vi "Clear All Disconnected MHLC.vi"(8 "error in (no error)":errorcluster, 10 "Data in":variant, 11 "AppMgr in":refnum<class "Application Manager.lvclass">) -> (0 "error out":errorcluster, 3 "AppMgr out":refnum<class "Application Manager.lvclass">)   [LabVIEW 2017, in "Application Manager.lvclass"]
doc: "Clear all disconnected applications from the tree"
uses:
  Application Manager.lvclass
  Application Manager.lvclass/Application Manager.ctl
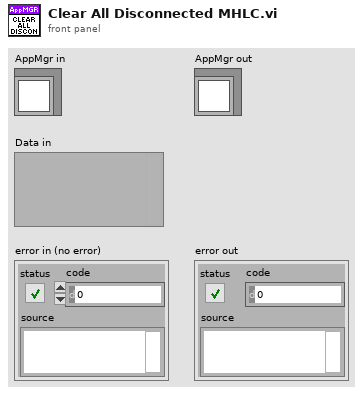
[diagram p1: front panel]
types:
  T1 = typedef "Application Manager.lvclass/Debug Client Data.ctl" = cluster{"DC_UID":T2, "IP Address":string, "Worker Data":T3[], "Connected":bool}
  T2 = typedef "DC_UID.ctl" = string
  T3 = typedef "Application Manager.lvclass/Worker Data.ctl" = cluster{"ID":string, "VI Ref":refnum<vi>, "VI Path":path, "CloneID":string, "Type":T4, "Worker Status":string}
  T4 = typedef "Workers.lvlib/Worker.lvclass/Worker Type.ctl" = enum16{"SL", "DL"}
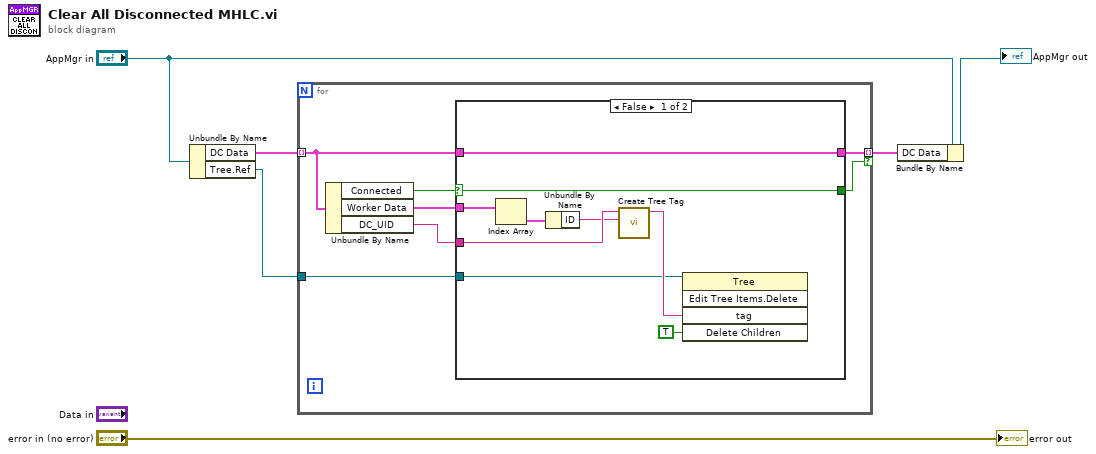
[diagram p0: block diagram]
diagram:
  n1 = Unbundle By Name("AppMgr in") -> ("DC Data"=w3:T1[], "Tree.Ref"=w4:refnum<vi>)
  n2 = for {
    tunnel: w4 -> [w11]
    tunnel: w3 -> [w8] mode=indexing
    tunnel: [w10] -> w2 mode=indexing if=w7
    n3 = Unbundle By Name(w8) -> ("Connected"=w9:bool, "Worker Data"=w12:T3[], "DC_UID"=w13:T2)
    n4 = case shown="False" w9 {
      selector: w9 -> [w15 w24]
      tunnel: w13 -> [w20 _]
      tunnel: w12 -> [w22 _]
      tunnel: w11 -> [w17 _]
      tunnel: w8 -> [w16 w23]
      tunnel: [w16 w23] -> w10
      tunnel: [w15 w24] -> w7
      frame False {
        n5 = Index Array(array=w22) -> (element=w21:T3)  [unwired: 1 in]
        n6 = Unbundle By Name(w21) -> ("ID"=w19:string)
        n7 = call "Create Tree Tag.vi"("WID"=w19, "DC_UID"=w20) -> ("Tree Tag"=w18:string)  [unwired: 9 in]
        n8 = invoke class="Tree" method="Edit Tree Items.Delete"(reference=w17, "tag"=w18, "Delete Children"=TRUE ("Delete Children?")) -> ()  [unwired: 2 in, 5 out]
      }
      frame True {
      }
    }
  }
  n9 = Bundle By Name(cluster="AppMgr in", "DC Data"=w2) -> (→"AppMgr out":refnum<class "Application Manager.lvclass">)
  "error out" <- "error in (no error)"
